vi "spec.vi"(11 "format (%.3f)":string="%.3f" caption="格式(%.3f)") -> (3 "first row":dbl[](array[numeric]) caption="第一行" format="%0.3f")   [LabVIEW 2011]
uses:
  <vilib>/Utility/file.llb/Read From Spreadsheet File (DBL).vi
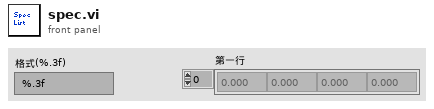
[diagram p1: front panel]
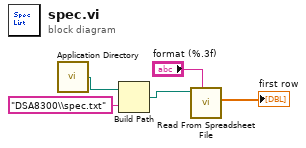
[diagram p0: block diagram]
diagram:
  n1 = call <vilib>:"Application Directory.vi"() -> ("Application Directory"=w5:path)
  n2 = Build Path(base path=w5, name or relative path="DSA8300\\spec.txt" ("名称或相对路径")) -> (appended path=w3:path)
  n3 = call-poly <vilib>:"Read From Spreadsheet File.vi"("format (%.3f)"="format (%.3f)", "file path (dialog if empty)"=w3) -> ("first row"=→"first row":dbl[])  [unwired: 5 in, 4 out]
